vi "SWERVE_DRIVE_MODULE_ACQUIRE.vi"(8 "Pass_Through_Time":dbl=-1.0 format="%33.4f", 11 "Swerve Module TypDef":T4) -> (0 "Swerve Rotational Speed Rad/Sec":dbl, 1 "Swerve Rel Angle Rad":dbl, 2 "Wheel Speed  M/S":dbl, 3 "Wheel Distance  M":dbl, 4 "Swerve Rel Rotation  Rad":T2 {"SIN" format="%13.4f"; "COS" format="%13.4f"; "VALUE" format="%13.4f"}, 5 "Swerve Module State":T3={"Speed"=0.0, "Angle"={"VALUE"=0.0, "COS"=1.0, "SIN"=0.0}} {"Angle"."SIN" format="%13.4f"; "Angle"."COS" format="%13.4f"; "Angle"."VALUE" format="%13.4f"}, 6 "SWERVE DRIVE MODULE POSITION":T1={"Distance"=0.0, "Angle"={"VALUE"=0.0, "COS"=1.0, "SIN"=0.0}, "P"=FALSE} {"Angle"."SIN" format="%13.4f"; "Angle"."COS" format="%13.4f"; "Angle"."VALUE" format="%13.4f"})   [LabVIEW 2019]
uses:
  SWERVE_DRIVE_MODULE_TYPDEF.ctl
  <vilib>/Rock Robotics/WPI/MotorControl/WPI_MotorControlDeviceRef.ctl
  <vilib>/Rock Robotics/WPI/MotorControl/WPI_MotorControlType.ctl
  <vilib>/Rock Robotics/SystemInterfaces/DIO/FPGA_DIOPWMChannel.ctl
  <vilib>/Rock Robotics/WPI/PWM/WPI_PWMDeadband.ctl
  <vilib>/Rock Robotics/SystemInterfaces/DIO/FPGA_DIOChannel.ctl
  <vilib>/Rock Robotics/WPI/Encoder/WPI_EncoderDevRef.ctl
  <vilib>/Rock Robotics/SystemInterfaces/Encoder/FPGA_EncoderIdx.ctl
  <vilib>/Rock Robotics/SystemInterfaces/Counter/FPGA_CounterCtrSystemIndex.ctl
  <vilib>/Rock Robotics/WPI/Encoder/WPI_EncoderType.ctl
  <vilib>/Rock Robotics/WPI/ThirdParty/JAS_Junk/TrajLib/TypeDef/ROTATION2D.ctl
  <vilib>/Rock Robotics/WPI/ThirdParty/JAS_Junk/TrajLib/TypeDef/SWERVE_DRIVE_MODULE_STATE.ctl
  <vilib>/Rock Robotics/WPI/ThirdParty/JAS_Junk/TrajLib/TypeDef/SWERVE_DRIVE_MODULE_POSITION.ctl
  <vilib>/Rock Robotics/WPI/ThirdParty/JAS_Junk/TrajLib/MathUtil_InputModulus.vi
  <vilib>/Rock Robotics/WPI/ThirdParty/JAS_Junk/TrajLib/Trajectory_Library.lvlib
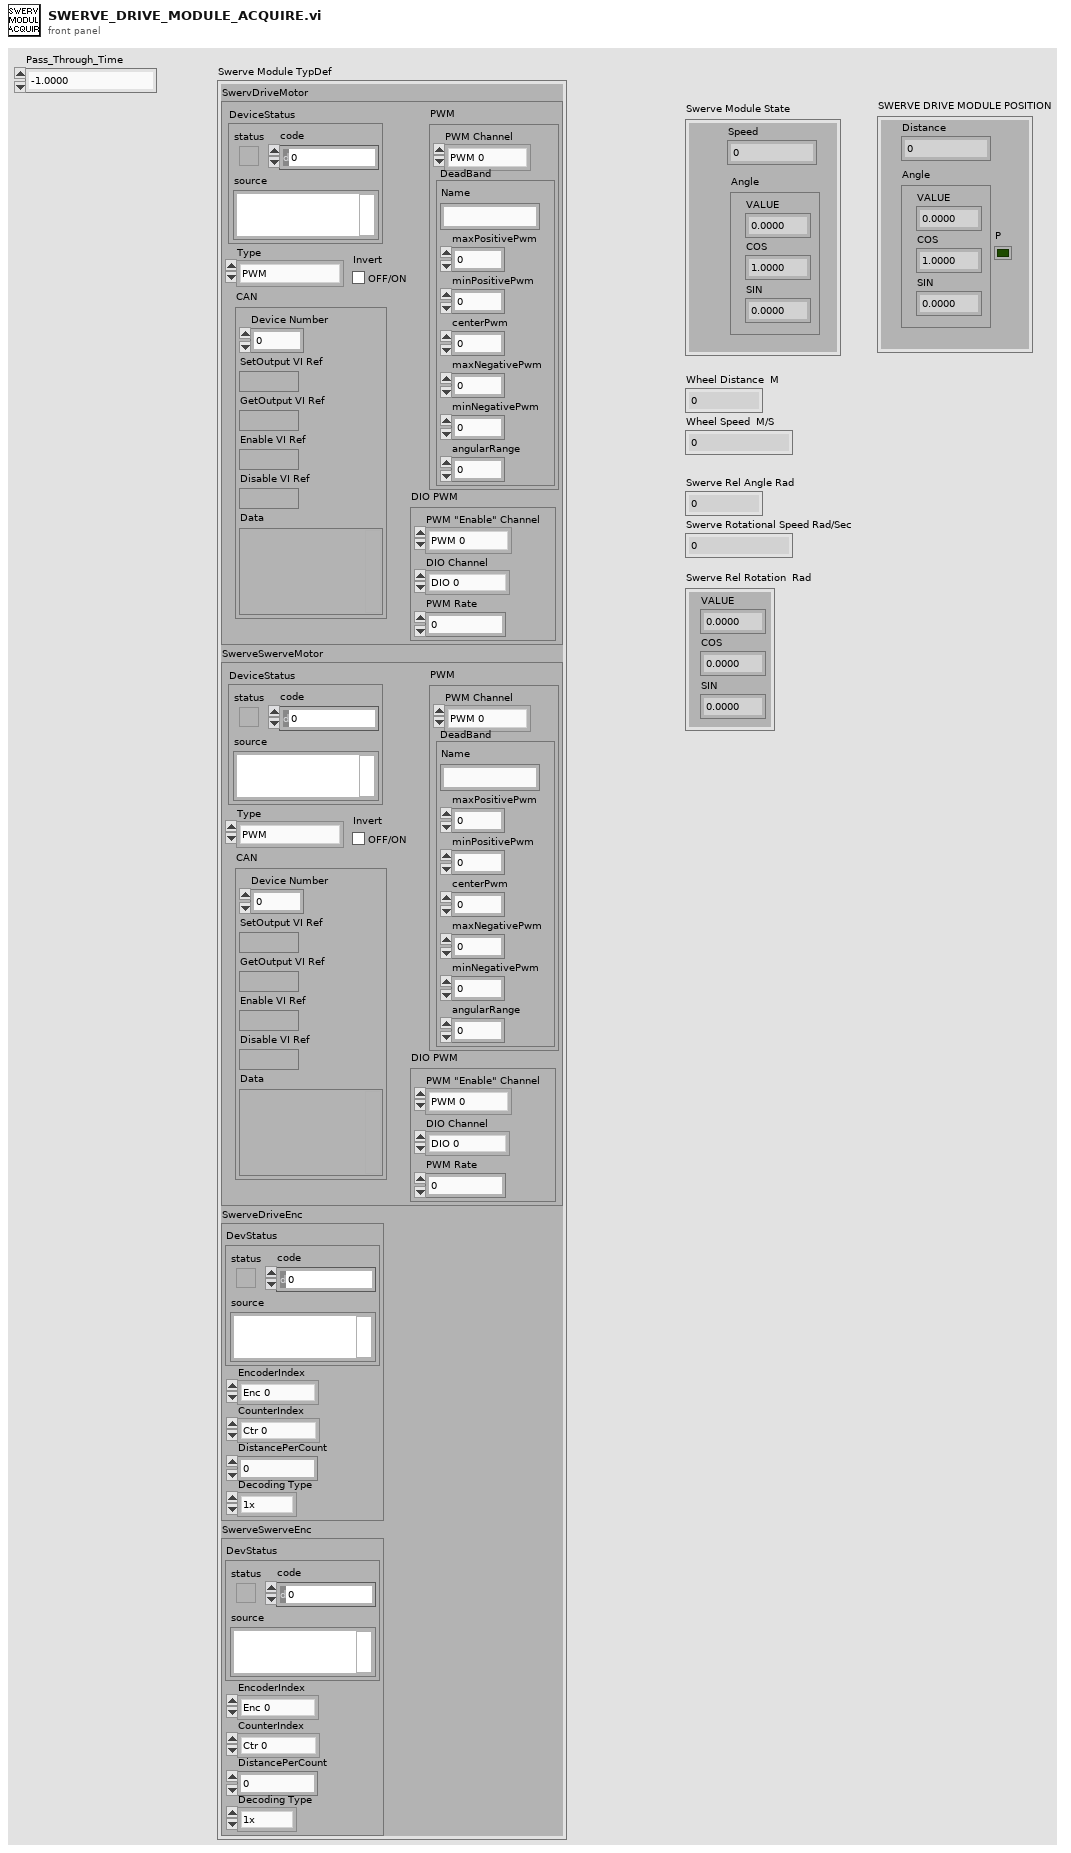
[diagram p1: front panel]
types:
  T1 = typedef "Trajectory_Library.lvlib/SWERVE_DRIVE_MODULE_POSITION.ctl" = cluster{"Distance":dbl, "Angle":T2, "P":bool}
  T2 = typedef "Trajectory_Library.lvlib/ROTATION2D.ctl" = cluster{"VALUE":dbl, "COS":dbl, "SIN":dbl}
  T3 = typedef "Trajectory_Library.lvlib/SWERVE_DRIVE_MODULE_STATE.ctl" = cluster{"Speed":dbl, "Angle":T2}
  T4 = typedef "SWERVE_DRIVE_MODULE_TYPDEF.ctl" = cluster{"SwervDriveMotor":T5, "SwerveSwerveMotor":T5, "SwerveDriveEnc":T10, "SwerveSwerveEnc":T10}
  T5 = typedef "WPI_MotorControlDeviceRef.ctl" = cluster{"DeviceStatus":errorcluster, "Type":T6, "PWM":cluster{"PWM Channel":T7, "DeadBand":T8}, "CAN":cluster{"Device Number":u8, "SetOutput VI Ref":variant, "GetOutput VI Ref":variant, "Enable VI Ref":variant, "Disable VI Ref":variant, "Data":variant}, "Invert":bool, "DIO PWM":cluster{"PWM \"Enable\" Channel":T7, "DIOChannel":T9, "PWM Rate":dbl}}
  T6 = typedef "WPI_MotorControlType.ctl" = enum16{"PWM", "CAN", "DIO PWM"}
  T7 = typedef "FPGA_DIOPWMChannel.ctl" = enum8{"PWM 0", "PWM 1", "PWM 2", "PWM 3", "PWM 4", "PWM 5", "PWM 6", "PWM 7", "PWM 8", "PWM 9", "PWM MXP 0", "PWM MXP 1", "PWM MXP 2", "PWM MXP 3", "PWM MXP 4", "PWM MXP 5", "PWM MXP 6", "PWM MXP 7", "PWM MXP 8", "PWM MXP 9", "Invalid"}
  T8 = typedef "WPI_PWMDeadband.ctl" = cluster{"Name":string, "maxPositivePwm":i32, "minPositivePwm":i32, "centerPwm":i32, "maxNegativePwm":i32, "minNegativePwm":i32, "angularRange":u16}
  T9 = typedef "FPGA_DIOChannel.ctl" = enum8{"DIO 0", "DIO 1", "DIO 2", "DIO 3", "DIO 4", "DIO 5", "DIO 6", "DIO 7", "DIO 8", "DIO 9", "DIO MXP 0", "DIO MXP 1", "DIO MXP 2", "DIO MXP 3", "DIO MXP 4", "DIO MXP 5", "DIO MXP 6", "DIO MXP 7", "DIO MXP 8", "DIO MXP 9", "DIO MXP 10", "DIO MXP 11", "DIO MXP 12", "DIO MXP 13", "DIO MXP 14", "DIO MXP 15", "SPI Port CS1", "SPI Port CS2", "SPI Port CS3", "SPI Port MISO", "SPI Port MOSI", "Invalid"}
  T10 = typedef "WPI_EncoderDevRef.ctl" = cluster{"DevStatus":errorcluster, "EncoderIndex":T11, "CounterIndex":T12, "DistancePerCount":dbl, "Decoding Type":T13}
  T11 = typedef "FPGA_EncoderIdx.ctl" = enum8{"Enc 0", "Enc 1", "Enc 2", "Enc 3", "Enc 4", "Enc 5", "Enc 6", "Enc 7", "Invalid"}
  T12 = typedef "FPGA_CounterCtrSystemIndex.ctl" = enum8{"Ctr 0", "Ctr 1", "Ctr 2", "Ctr 3", "Ctr 4", "Ctr 5", "Ctr 6", "Ctr 7", "Invalid"}
  T13 = typedef "WPI_EncoderType.ctl" = enum16{"1x", "2x", "4x"}
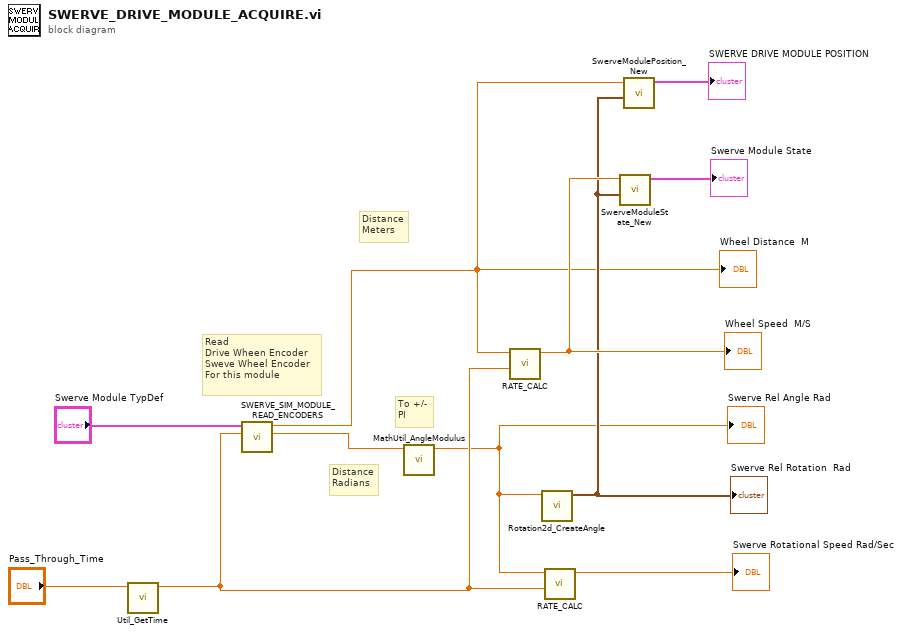
[diagram p0: block diagram]
diagram:
  # "Read \nDrive Wheen Encoder\nSweve Wheel Encoder\nFor this module"
  # "Distance\nRadians"
  # "Distance\nMeters"
  # "To +/-\nPI"
  n1 = call <vilib>:"Util_GetTime.vi"("Pass_Through_Time"="Pass_Through_Time") -> ("FPGA_Time_Seconds"=w4:dbl)  [unwired: 9 in, 1 out]
  n2 = call "SWERVE_SIM_MODULE_READ_ENCODERS.vi"("FPGA_Time_Seconds"=w4, "Swerve Module TypDef"="Swerve Module TypDef") -> ("Swerve Distance_Radians"=w2:dbl, "Wheel Distance_Meters"=w1:dbl)  [unwired: 8 in]
  "Wheel Distance  M" <- w1
  n3 = call <vilib>:"MathUtil_AngleModulus.vi"("InputAngle"=w2) -> ("ModulsAngle"=w3:dbl)  [unwired: 10 in]
  "Swerve Rel Angle Rad" <- w3
  n4 = call "RATE_CALC.vi"("Time"=w4, "Input"=w1) -> ("Output"=w9:dbl)  [unwired: 9 in]
  "Wheel Speed  M/S" <- w9
  n5 = call <vilib>:"Rotation2d_CreateAngle.vi"("Angle"=w3) -> ("ROTATION"=w7:T2)  [unwired: 10 in]
  "Swerve Rel Rotation  Rad" <- w7
  n6 = call "RATE_CALC.vi"("Time"=w4, "Input"=w3) -> ("Output"=→"Swerve Rotational Speed Rad/Sec":dbl)  [unwired: 9 in]
  n7 = call <vilib>:"SwerveModuleState_New.vi"("ROTATION"=w7, "Speed"=w9) -> ("SWERVE_DRIVE_MODULE_STATE"=→"Swerve Module State":T3)  [unwired: 9 in]
  n8 = call <vilib>:"SwerveModulePosition_New.vi"("ROTATION"=w7, "Distance"=w1) -> ("SWERVE_DRIVE_MODULE_POSITION"=→"SWERVE DRIVE MODULE POSITION":T1)  [unwired: 9 in]
